vi "TTA_MXG_ARB.vi"(0 "VISA resource In":refnum<visa-resource-name>, 1 "Waveform File":string="ON", 5 "Frequency (MHz)":dbl, 7 "Output Power\nLevel (dBm)":dbl, 9 "ARB Sample Rate":dbl, 11 "error in":errorcluster) -> (4 "VISA resource Out":refnum<visa-resource-name>, 15 "error out":errorcluster)   [LabVIEW 2016]
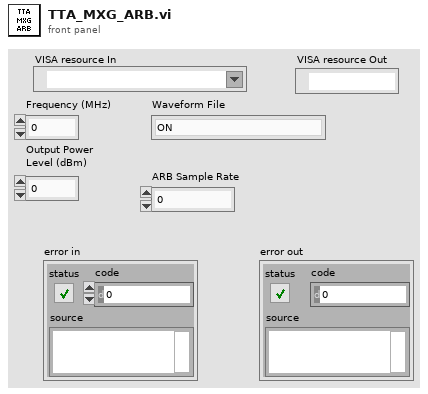
[diagram p1: front panel]
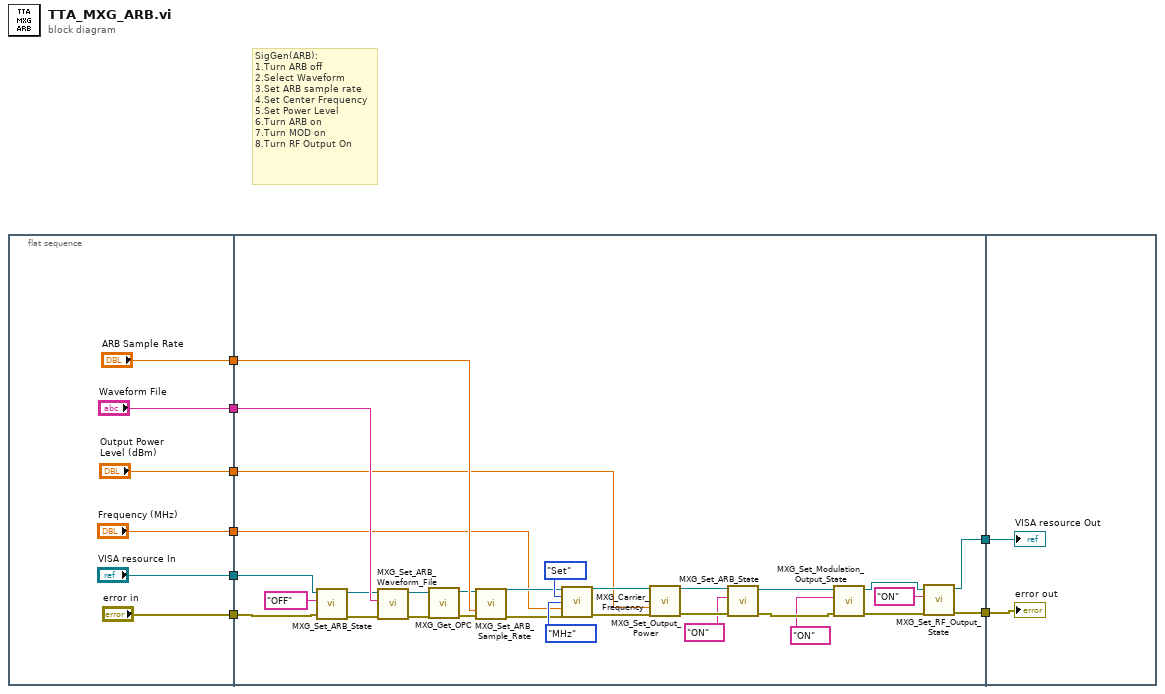
[diagram p0: block diagram]
diagram:
  # "SigGen(ARB):\n1.Turn ARB off\n2.Select Waveform\n3.Set ARB sample rate\n4.Set Center Frequency\n5.Set Power Level\n6.Turn ARB on\n7.Turn MOD on\n8.Turn RF Output On"
  n1 = flat-sequence {
    tunnel: ["error in"] -> w8
    tunnel: ["VISA resource In"] -> w7
    tunnel: ["Frequency (MHz)"] -> w6
    tunnel: ["Output Power\nLevel (dBm)"] -> w5
    tunnel: ["Waveform File"] -> w4
    tunnel: ["ARB Sample Rate"] -> w3
    tunnel: w8 -> [w43]
    tunnel: w7 -> [w42]
    tunnel: w6 -> [w31]
    tunnel: w5 -> [w30]
    tunnel: w4 -> [w40]
    tunnel: w3 -> [w38]
    tunnel: [w20] -> w2
    tunnel: [w19] -> w1
    tunnel: w2 -> [w46]
    tunnel: w1 -> [w45]
    frame #0 {
    }
    frame #1 {
      n2 = call "MXG_Set_ARB_State.vi"("error in"=w43, "ARB State"="OFF", "VISA resource name"=w42) -> ("error out"=w41:errorcluster, "VISA resource name"=w39:refnum<visa-resource-name>)  [unwired: 7 in]
      n3 = call "MXG_Set_ARB_Waveform_File.vi"("error in"=w41, "Waveform File"=w40, "VISA resource name"=w39) -> ("error out"=w18:errorcluster, "VISA resource name"=w17:refnum<visa-resource-name>)  [unwired: 7 in]
      n4 = call "MXG_Get_OPC.vi"("error in"=w18, "VISA resource name"=w17) -> ("error out"=w15:errorcluster, "VISA resource name"=w16:refnum<visa-resource-name>)  [unwired: 7 in, 1 out]
      n5 = call "MXG_Set_ARB_Sample_Rate.vi"("VISA resource name"=w16, "ARB Sample Rate"=w38, "error in"=w15) -> ("VISA resource name"=w34:refnum<visa-resource-name>, "error out"=w35:errorcluster)  [unwired: 11 in]
      n6 = call "MXG_Carrier_Frequency.vi"("VISA resource name"=w34, "Mode"=enum16{"Set", "Get"}."Set", "Units"=enum16{"Hz", "kHz", "MHz", "GHz"}."MHz", "Frequency"=w31, "error in"=w35) -> ("VISA resource name"=w32:refnum<visa-resource-name>, "error out"=w33:errorcluster)  [unwired: 8 in, 1 out]
      n7 = call "MXG_Set_Output_Power.vi"("VISA resource name"=w32, "Output Power\nLevel (dBm)"=w30, "error in"=w33) -> ("VISA resource name"=w28:refnum<visa-resource-name>, "error out"=w29:errorcluster)  [unwired: 11 in]
      n8 = call "MXG_Set_ARB_State.vi"("error in"=w29, "ARB State"="ON", "VISA resource name"=w28) -> ("error out"=w26:errorcluster, "VISA resource name"=w24:refnum<visa-resource-name>)  [unwired: 7 in]
      n9 = call "MXG_Set_Modulation_Output_State.vi"("error in"=w26, "Modulation State"="ON", "VISA resource name"=w24) -> ("error out"=w21:errorcluster, "VISA resource name"=w22:refnum<visa-resource-name>)  [unwired: 7 in]
      n10 = call "MXG_Set_RF_Output_State.vi"("error in"=w21, "RF Output State"="ON", "VISA resource name"=w22) -> ("error out"=w20:errorcluster, "VISA resource name"=w19:refnum<visa-resource-name>)  [unwired: 7 in]
    }
    frame #2 {
      "VISA resource Out" <- w45
      "error out" <- w46
    }
  }
